vi "Menu.vi"() -> ()   [LabVIEW 2021]
panel:
  out "error out":errorcluster
  in  "error in":errorcluster
  out "String":string
  in  "Exit":bool
  out "Access":bool
  in  "Cluster":T1
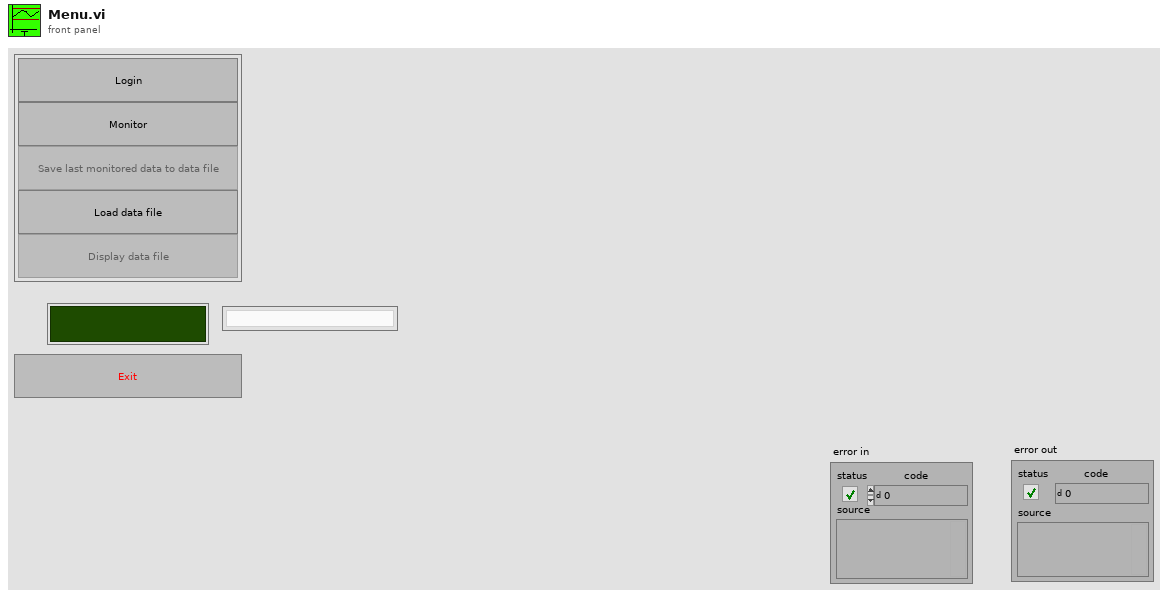
[diagram p1: front panel]
types:
  T1 = cluster{"Login button":bool, "Monitor button":bool, "Save data button":bool, "Load data button":bool, "Display data button":bool}
  T2 = enum8{"Enabled", "Disabled", "Disabled and Grayed Out"}
  T3 = enum16{"open", "replace", "create", "open or create", "replace or create", "replace or create with confirmation"}
  T4 = cluster{"User Name output":string, "Time/Date":timestamp, "Datos Finales":cluster{"Temp.Max":dbl, "Temp.Actual":dbl, "Temp.Min":dbl}[]}
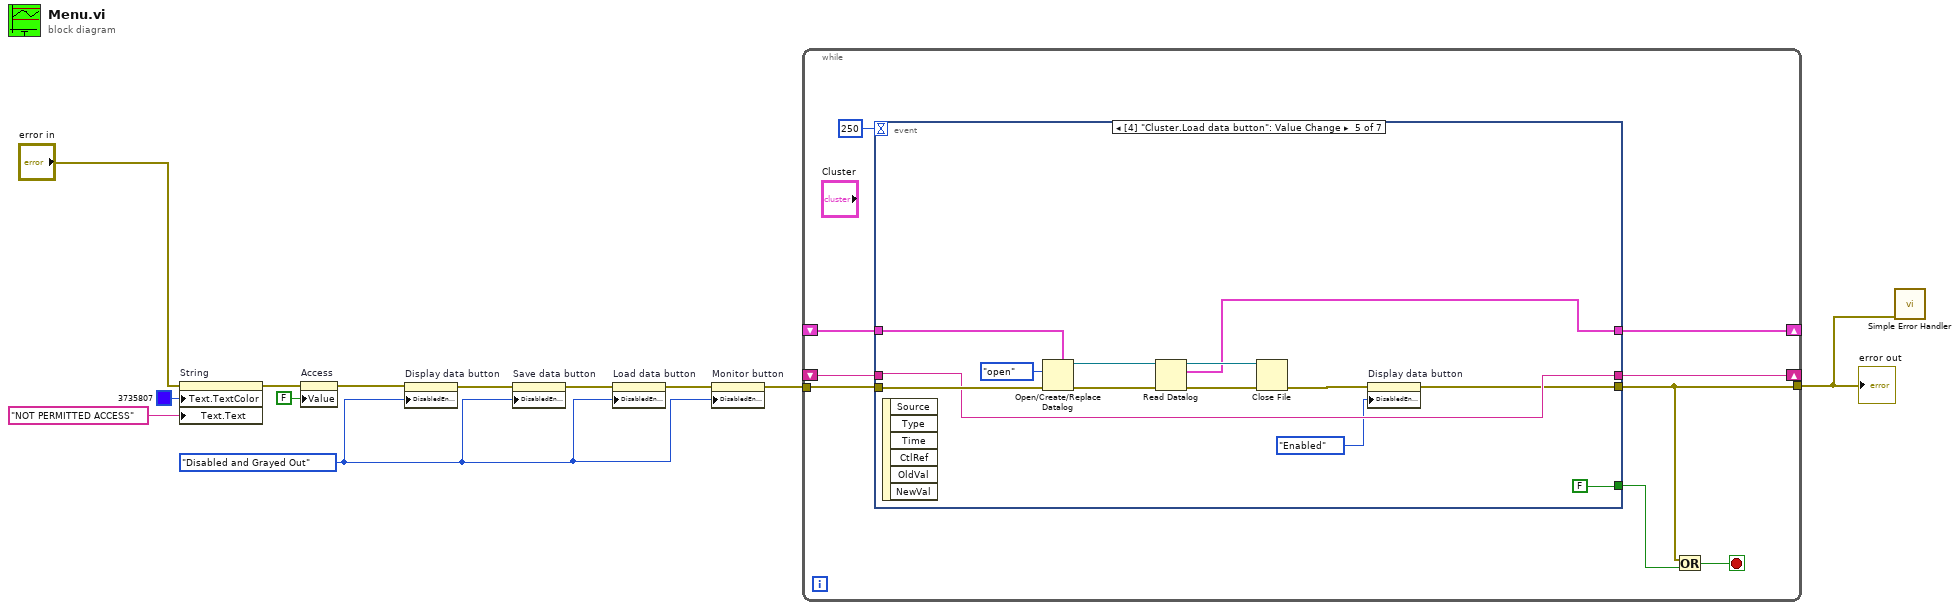
[diagram p0: block diagram]
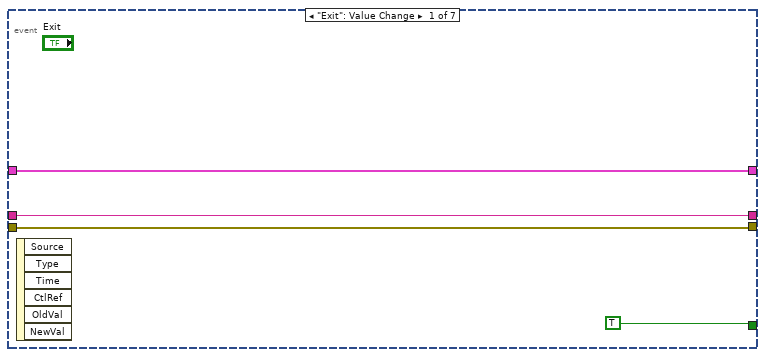
[diagram p2: hidden frame]
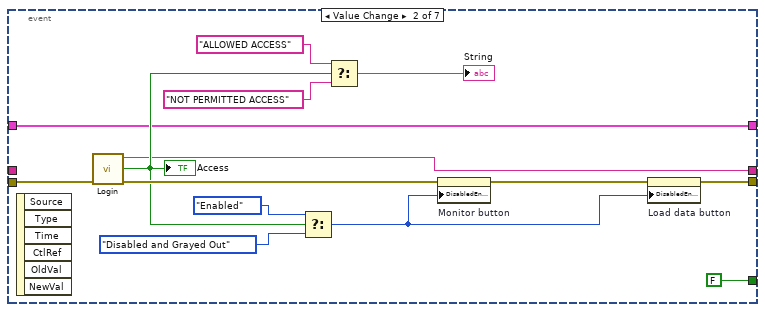
[diagram p3: hidden frame]
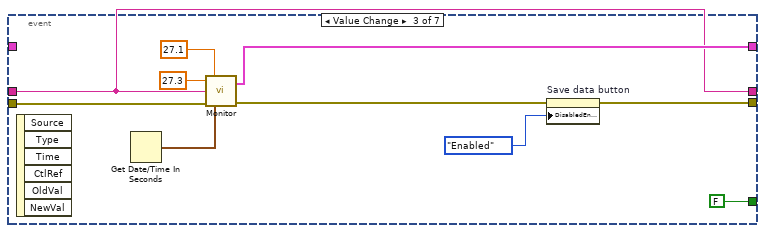
[diagram p4: hidden frame]
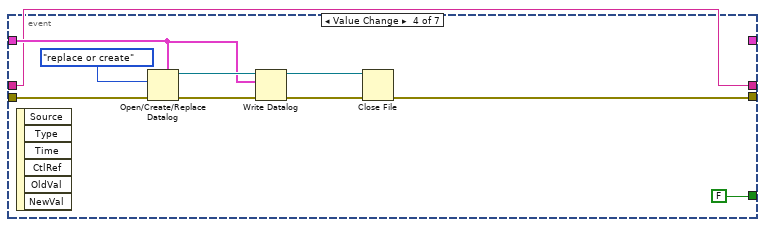
[diagram p5: hidden frame]
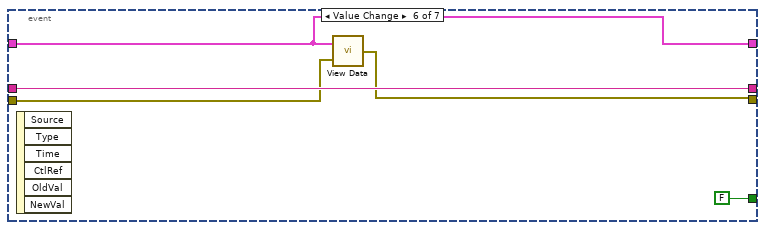
[diagram p6: hidden frame]
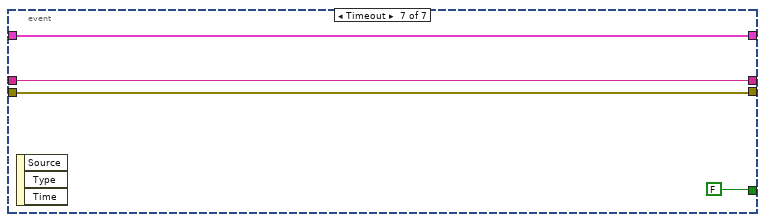
[diagram p7: hidden frame]
diagram:
  w8 = T2."Disabled and Grayed Out" ("Disabled")
  n1 = property on="String" class="Str"(error in="error in", "Text.TextColor"=u32 3735807 ("Text.Text Colors:Text Color"), "Text.Text"="NOT PERMITTED ACCESS") -> (error out=w4:errorcluster)  [unwired: 1 in, 1 out]
  n2 = property on="Access" class="Bool (strict)"(error in=w4, "Value"=FALSE ("Access")) -> (error out=w7:errorcluster)  [unwired: 1 in, 1 out]
  n3 = property on="Display data button" class="Bool"(error in=w7, "DisabledEnum"=w8) -> (error out=w12:errorcluster)  [unwired: 1 in, 1 out]
  n4 = property on="Save data button" class="Bool"(error in=w12, "DisabledEnum"=w8) -> (error out=w11:errorcluster)  [unwired: 1 in, 1 out]
  n5 = property on="Load data button" class="Bool"(error in=w11, "DisabledEnum"=w8) -> (error out=w9:errorcluster)  [unwired: 1 in, 1 out]
  n6 = property on="Monitor button" class="Bool"(error in=w9, "DisabledEnum"=w8) -> (error out=w10:errorcluster)  [unwired: 1 in, 1 out]
  n7 = while {
    tunnel: [w19] -> w1
    tunnel: w10 -> [w20]
    shift-right: [w16] -> _
    shift-left: _ -> [w15]
    shift-right: [w14] -> _
    shift-left: _ -> [w13]
    stop <- w17 stop-if-true
    n8 = event shown="[4] \"Cluster.Load data button\": Value Change" {
      selector: _ -> [_ _ _ _ _ _ _]
      dyn-events: _ -> [_ _ _ _ _ _ _]
      timeout: 250 -> [_ _ _ _ _ _ _]
      tunnel: [TRUE FALSE FALSE FALSE FALSE FALSE FALSE] -> w18
      tunnel: [w24 w36 w48 w50 w60 w74 w81] -> w19
      tunnel: w20 -> [w24 w38 w44 w54 w68 w75 w81]
      tunnel: [w22 w28 w40 w51 w63 w76 w79] -> w16
      tunnel: w15 -> [w22 _ w40 w51 w63 w76 w79]
      tunnel: [w23 w26 w41 _ w65 w73 w78] -> w14
      tunnel: w13 -> [w23 w26 _ w52 w71 w73 w78]
      event "Exit": Value Change {
        n9 = event-data() -> ()  [unwired: 1 in, 6 out]
      }
      event "Cluster.Login button": Value Change {
        n10 = event-data() -> ()  [unwired: 1 in, 6 out]
        n11 = call "Login.vi"("error in (no error)"=w38) -> ("error out"=w37:errorcluster, "Access"=w29:bool, "User"=w28:string)  [unwired: 4 in]
        "Access" <- w29
        n12 = Select(t=T2."Enabled" ("Disabled"), s=w29, f=T2."Disabled and Grayed Out" ("Disabled")) -> (s? t:f=w33:T2)
        n13 = Select(t="ALLOWED ACCESS", s=w29, f="NOT PERMITTED ACCESS") -> (s? t:f=→"String":string)
        n14 = property on="Monitor button" class="Bool"(error in=w37, "DisabledEnum"=w33) -> (error out=w27:errorcluster)  [unwired: 1 in, 1 out]
        n15 = property on="Load data button" class="Bool"(error in=w27, "DisabledEnum"=w33) -> (error out=w36:errorcluster)  [unwired: 1 in, 1 out]
      }
      event "Cluster.Monitor button": Value Change {
        n16 = event-data() -> ()  [unwired: 1 in, 6 out]
        n17 = Get Date/Time In Seconds() -> (seconds since 1Jan1904=w43:timestamp)
        n18 = call "Monitor.vi"("Temp.Max"=27.3, "Temp.Min"=27.1, "User name input"=w40, "error in (no error)"=w44, "Time/Date"=w43) -> ("History Data"=w41:T4, "error out"=w42:errorcluster)
        n19 = property on="Save data button" class="Bool"(error in=w42, "DisabledEnum"=T2."Enabled" ("Disabled")) -> (error out=w48:errorcluster)  [unwired: 1 in, 1 out]
      }
      event "Cluster.Save data button": Value Change {
        n20 = event-data() -> ()  [unwired: 1 in, 6 out]
        n21 = Open/Create/Replace Datalog(5:w52, 8:w54, 10:T3."replace or create" ("operation (0:open)")) -> (0:w56:errorcluster, 3:w58:refnum<k1>)  [unwired: 3 in, 1 out]
        n22 = Write Datalog(4:w56, 6:w52, 7:w58) -> (0:w55:errorcluster, 3:w57:refnum<k1>)
        n23 = Close File(refnum=w57, error in=w55) -> (error out=w50:errorcluster)  [unwired: 1 out]
      }
      event "Cluster.Load data button": Value Change {
        n24 = event-data() -> ()  [unwired: 1 in, 6 out]
        n25 = Open/Create/Replace Datalog(5:w71, 8:w68, 10:T3."open" ("operation (0:open)")) -> (0:w67:errorcluster, 3:w70:refnum<k1>)  [unwired: 3 in, 1 out]
        n26 = Read Datalog(4:w67, 7:w70) -> (0:w66:errorcluster, 2:w65:T4, 3:w69:refnum<k1>)  [unwired: 1 in]
        n27 = Close File(refnum=w69, error in=w66) -> (error out=w61:errorcluster)  [unwired: 1 out]
        n28 = property on="Display data button" class="Bool"(error in=w61, "DisabledEnum"=T2."Enabled" ("Disabled")) -> (error out=w60:errorcluster)  [unwired: 1 in, 1 out]
      }
      event "Cluster.Display data button": Value Change {
        n29 = event-data() -> ()  [unwired: 1 in, 6 out]
        n30 = call "View Data.vi"("error in (no error)"=w75, "Historic Data Input"=w73) -> ("error out"=w74:errorcluster)
      }
      event Timeout {
        n31 = event-data() -> ()  [unwired: 1 in, 3 out]
      }
    }
    n32 = Or(x=w19, y=w18) -> (x .or. y?=w17:bool)
  }
  "error out" <- w1
  n33 = call <vilib>:"Simple Error Handler.vi"("error in (no error)"=w1) -> ()  [unwired: 4 in, 5 out]
